vi "TDMS_write.vi"() -> ()   [LabVIEW 2012]
panel:
  in  "Data":dbl[](array[numeric])
  in  "Size Y":dbl
  in  "Size X":dbl
  in  "Frequency":dbl
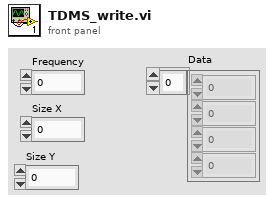
[diagram p1: front panel]
types:
  T1 = enum16{"open", "open or create", "create or replace", "create", "open (read-only)"}
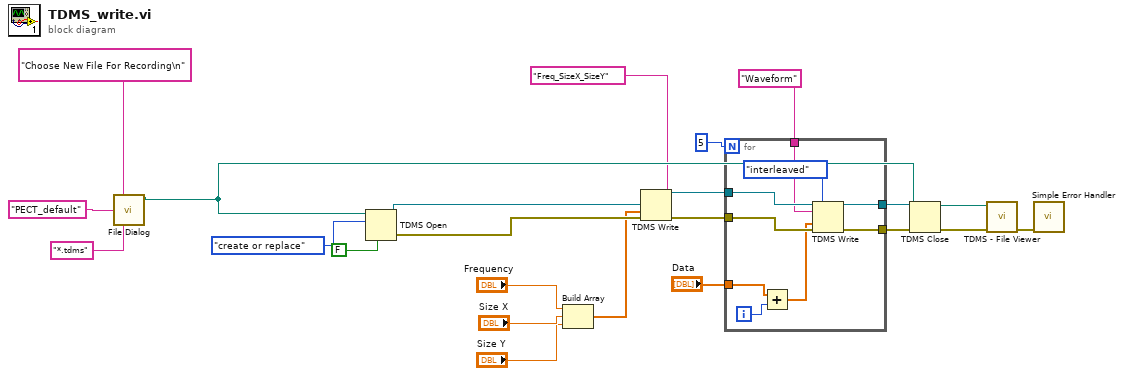
[diagram p0: block diagram]
diagram:
  n1 = call "File Dialog"("prompt"="Choose New File For Recording\n" ("button label"), "default name"="PECT_default", "pattern (all files)"="*.tdms") -> ("selected path"=w9:path)  [unwired: 9 in, 3 out]
  n2 = TDMS Open(6:FALSE ("disable buffering (T)"), 10:T1."create or replace" ("operation"), 11:w9) -> (0:w18:errorcluster, 3:w19:refnum<k34>)  [unwired: 3 in]
  n3 = Build Array("Frequency", "Size X", "Size Y") -> (w2:dbl[])
  n4 = TDMS Write(0:w19, 5:"Freq_SizeX_SizeY" ("group name in (Untitled)"), 9:w2, 11:w18) -> (4:w16:refnum<k34>, 15:w15:errorcluster)  [unwired: 2 in, 2 out]
  n5 = for {
    N: 5 -> [_]
    tunnel: w16 -> [w31]
    tunnel: w15 -> [w30]
    tunnel: [w29] -> w14
    tunnel: [w28] -> w13
    tunnel: "Waveform" ("group name in (Untitled)") -> [w27]
    tunnel: "Data" -> [w26]
    i -> [w23]
    n6 = Add(x=w26, y=w23) -> (x+y=w25:dbl[])
    n7 = TDMS Write(0:w31, 1:enum16{"decimated", "interleaved"}."interleaved" ("data layout (0:decimated)"), 5:w27, 9:w25, 11:w30) -> (4:w29:refnum<k34>, 15:w28:errorcluster)  [unwired: 1 in, 2 out]
  }
  n8 = TDMS Close(8:w13, 11:w14) -> (0:w22:errorcluster)  [unwired: 1 out]
  n9 = call <vilib>:"TDMS - File Viewer.vi"("error in (no error)"=w22, "file path"=w9) -> ("error out"=w21:errorcluster)  [unwired: 5 out]
  n10 = call <vilib>:"Simple Error Handler.vi"("error in (no error)"=w21) -> ()  [unwired: 1 in, 8 out]
